vi "EulerRotXYZ.vi"(11 "Euler Angle (XYZ)":dbl[](array[numeric])=[0.0, 0.0, 0.0]) -> (3 "Rotation Mtx":T1=[[1.0, 0.0, 0.0], [0.0, 1.0, 0.0], [0.0, 0.0, 1.0]])   [LabVIEW 2016]
uses:
  <vilib>/Analysis/Matrix/Datatypes/RealMatrix.ctl
  <vilib>/Analysis/baseanly.llb/Real A x B.vi
  <vilib>/Analysis/Matrix/Numeric/Conversions/Array To Matrix - RA2.vi
  <vilib>/Analysis/Matrix/NI_Matrix.lvlib
  <vilib>/Analysis/NI_AALBase.lvlib
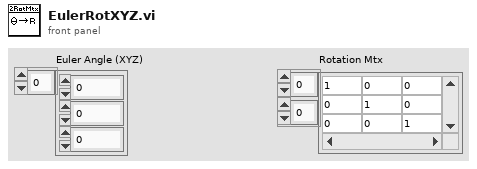
[diagram p1: front panel]
types:
  T1 = typedef "NI_Matrix.lvlib/RealMatrix.ctl" = dbl[][]
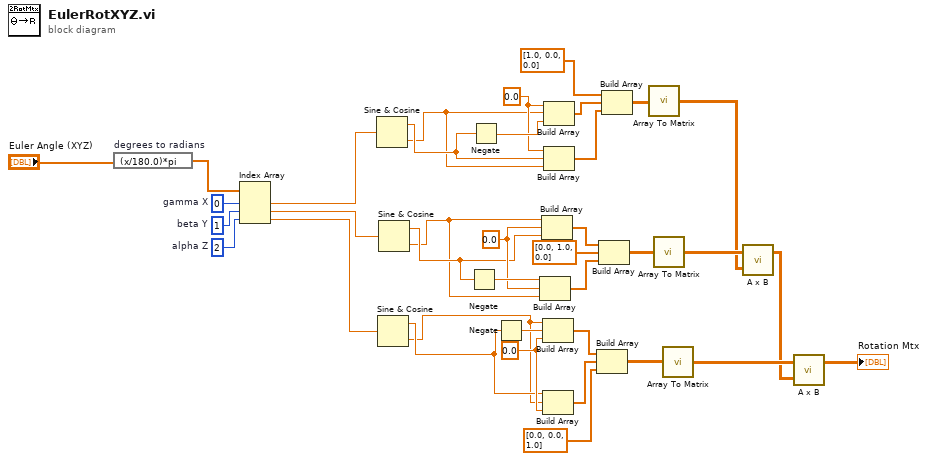
[diagram p0: block diagram]
diagram:
  w15 = 0.0 ("element")
  w21 = 0.0 ("element")
  w29 = 0.0 ("element")
  w33 = 2  # alpha Z
  w34 = 1  # beta Y
  w35 = 0  # gamma X
  n1 = expression code="(x/180.0)*pi" "degrees to radians"("Euler Angle (XYZ)") -> (w36:dbl[])
  n2 = Index Array(array=w36, index #1=w35, index #2=w34, index #3=w33) -> (element #1=w7:dbl, element #2=w6:dbl, element #3=w3:dbl)
  n3 = Sine & Cosine(0:w7) -> (1:w9:dbl, 2:w8:dbl)
  n4 = Sine & Cosine(0:w3) -> (1:w2:dbl, 2:w1:dbl)
  n5 = Sine & Cosine(0:w6) -> (1:w5:dbl, 2:w4:dbl)
  n6 = Negate(x=w5) -> (-x=w22:dbl)
  n7 = Negate(x=w9) -> (-x=w16:dbl)
  n8 = Negate(x=w2) -> (-x=w32:dbl)
  n9 = Build Array(w22, w21, w4) -> (w24:dbl[])
  n10 = Build Array(w4, w21, w5) -> (w25:dbl[])
  n11 = Build Array(w1, w32, w29) -> (w30:dbl[])
  n12 = Build Array(w2, w1, w29) -> (w31:dbl[])
  n13 = Build Array(w15, w8, w16) -> (w18:dbl[])
  n14 = Build Array(w15, w9, w8) -> (w17:dbl[])
  n15 = Build Array(w30, w31, dbl[] [0.0, 0.0, 1.0]) -> (w27:dbl[][])
  n16 = Build Array(w25, dbl[] [0.0, 1.0, 0.0], w24) -> (w20:dbl[][])
  n17 = Build Array(dbl[] [1.0, 0.0, 0.0], w18, w17) -> (w14:dbl[][])
  n18 = call-poly <vilib>:"Array To Matrix.vi"("Real 2D Array"=w14) -> ("Real Matrix"=w12:T1)
  n19 = call-poly <vilib>:"Array To Matrix.vi"("Real 2D Array"=w20) -> ("Real Matrix"=w13:T1)
  n20 = call-poly <vilib>:"Array To Matrix.vi"("Real 2D Array"=w27) -> ("Real Matrix"=w26:T1)
  n21 = call-poly <vilib>:"A x B.vi"("B"=w12, "A"=w13) -> ("A x B"=w11:T1)  [unwired: 1 out]
  n22 = call-poly <vilib>:"A x B.vi"("B"=w11, "A"=w26) -> ("A x B"=→"Rotation Mtx":T1)  [unwired: 1 out]
